vi "GetCtlValue_Core.vi"(8 "error in (no error)":errorcluster, 10 "CtlName In":string, 11 "CtlReferences in":refnum<class "CtlReferences.lvclass">) -> (0 "error out":errorcluster, 1 "Value":variant, 3 "CtlReferences out":refnum<class "CtlReferences.lvclass">)   [LabVIEW 2020, in "CtlReferences.lvlib" / "CtlReferences.lvclass"]
uses:
  CtlReferences.lvclass
  CtlReferences.lvclass/CtlReferences.ctl
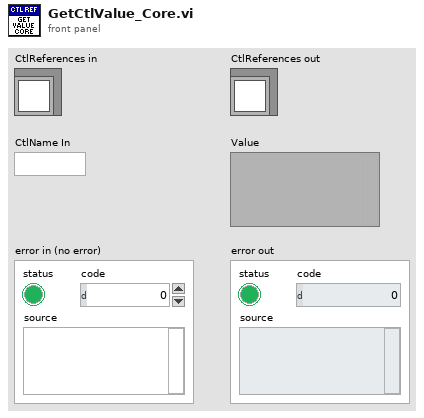
[diagram p1: front panel]
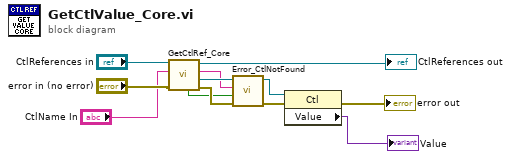
[diagram p0: block diagram]
diagram:
  n1 = call-dynamic "GetCtlRef_Core.vi"("error in (no error)"="error in (no error)", "CtlName In"="CtlName In", "CtlReferences in"="CtlReferences in") -> ("error out"=w7:errorcluster, "Ctl Refnum"=w9:refnum<vi>, "CtlName out"=w8:string, "CtlReferences out"=→"CtlReferences out":refnum<class "CtlReferences.lvclass">, "Found"=w6:bool)  [unwired: 4 in]
  n2 = call "Error_CtlNotFound.vi"("error in (no error)"=w7, "Control Found?"=w6, "CtlName"=w8, "Control in"=w9) -> ("error out"=w5:errorcluster, "Control out"=w4:refnum<vi>)  [unwired: 6 in]
  n3 = property class="Ctl"(reference=w4, error in=w5) -> (error out=→"error out":errorcluster, "Value"=→"Value":variant)  [unwired: 1 out]
